vi "Image - Center and Zoom.vi"(8 "Error In":errorcluster, 10 "Image Data":T2, 11 "Pict Refnum":refnum<vi>) -> (0 "Error Out":errorcluster, 2 "Rect Out":T1, 3 "new picture":picture)   [LabVIEW 2020]
uses:
  <vilib>/picture/picture.llb/imagedata.ctl
  <vilib>/Utility/miscctls.llb/LVPointTypeDef.ctl
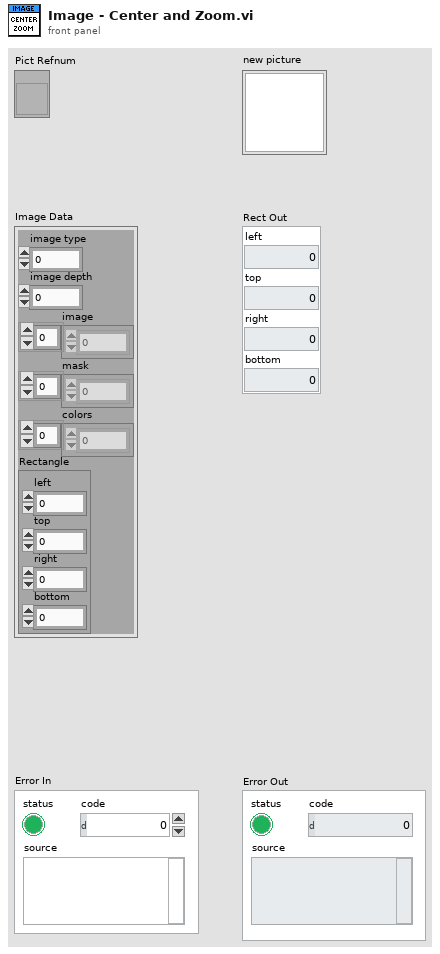
[diagram p1: front panel]
types:
  T1 = cluster{"left":i16, "top":i16, "right":i16, "bottom":i16}
  T2 = typedef "imagedata.ctl" = cluster{"image type":i32, "image depth":i32, "image":u8[], "mask":u8[], "colors":u32[], "Rectangle":cluster{"left":i16, "top":i16, "right":i16, "bottom":i16}}
  T3 = typedef "LVPointTypeDef.ctl" = cluster{"Horizontal":i16, "Vertical":i16}
  T4 = typedef "LVBoundsTypeDef.ctl" = cluster{"Width":u32, "Height":u32}
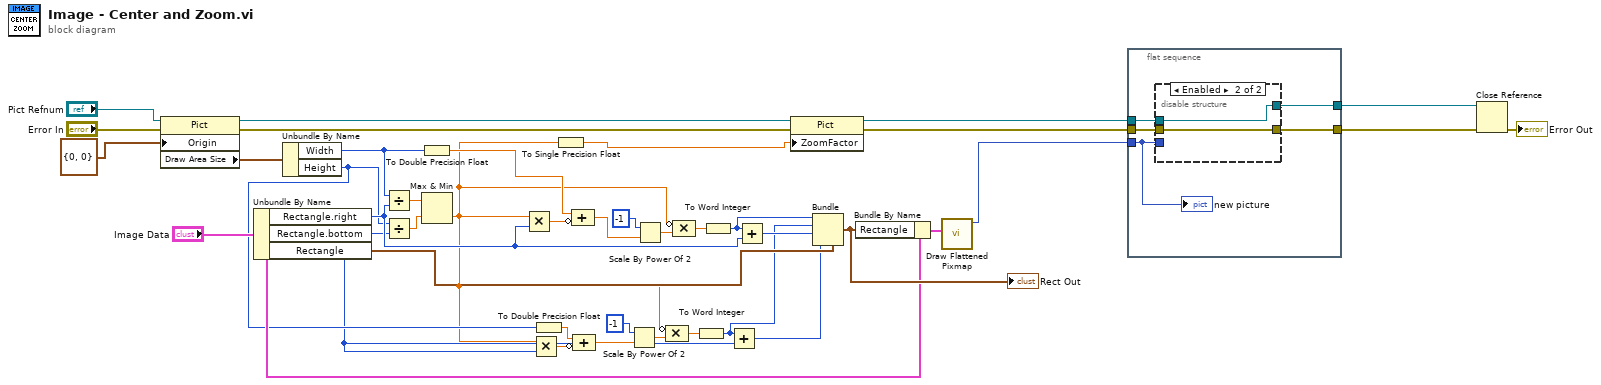
[diagram p0: block diagram]
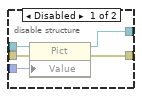
[diagram p2: hidden frame]
diagram:
  n1 = property class="Pict"(reference="Pict Refnum", error in="Error In", "Origin"=T3 {"Horizontal"=0, "Vertical"=0}) -> (reference out=w16:refnum<vi>, error out=w39:errorcluster, "Draw Area Size"=w17:T4)
  n2 = Unbundle By Name("Image Data") -> ("Rectangle.right"=w27:i16, "Rectangle.bottom"=w6:i16, "Rectangle"=w31:T1)
  n3 = Unbundle By Name(w17) -> ("Width"=w21:u32, "Height"=w7:u32)
  n4 = Divide(x=w21, y=w27) -> (x/y=w34:dbl)
  n5 = Divide(x=w7, y=w6) -> (x/y=w35:dbl)
  n6 = To Double Precision Float(number=w21) -> (double precision float=w32:dbl)
  n7 = Max & Min(x=w34, y=w35) -> (min(x,y)=w2:dbl)  [unwired: 1 out]
  n8 = Multiply(x=w2, y=w27) -> (x*y=w26:dbl)
  n9 = Multiply(x=w2, y=w6) -> (x*y=w13:dbl)
  n10 = To Double Precision Float(number=w7) -> (double precision float=w12:dbl)
  n11 = To Single Precision Float(number=w2) -> (single precision float=w1:sgl)
  n12 = Compound Arithmetic op=ADD(w32, invert w26) -> (w25:dbl)
  n13 = Compound Arithmetic op=ADD(w12, invert w13) -> (w8:dbl)
  n14 = Scale By Power Of 2(n=i16 -1, x=w8) -> (x*2^n=w10:dbl)
  n15 = Scale By Power Of 2(n=i16 -1, x=w25) -> (x*2^n=w24:dbl)
  n16 = Compound Arithmetic op=MULTIPLY(invert w2, w10) -> (w11:dbl)
  n17 = Compound Arithmetic op=MULTIPLY(invert w2, w24) -> (w23:dbl)
  n18 = To Word Integer(number=w11) -> (16bit integer=w5:i16)
  n19 = To Word Integer(number=w23) -> (16bit integer=w22:i16)
  n20 = Add(x=w5, y=w6) -> (x+y=w4:i16)
  n21 = Add(x=w22, y=w27) -> (x+y=w30:i16)
  n22 = property class="Pict"(reference=w16, error in=w39, "ZoomFactor"=w1) -> (reference out=w14:refnum<vi>, error out=w38:errorcluster)
  n23 = Bundle(cluster=w31, "left"=w22, "top"=w5, "right"=w30, "bottom"=w4) -> (w29:T1)
  "Rect Out" <- w29
  n24 = Bundle By Name(cluster="Image Data", "Rectangle"=w29) -> (w28:T2)
  n25 = call <vilib>:"Draw Flattened Pixmap.vi"("image data"=w28) -> ("new picture"=w15:picture)  [unwired: 8 in]
  n26 = flat-sequence {
    tunnel: w38 -> [w45]
    tunnel: [w44] -> w36
    tunnel: w15 -> [w41]
    tunnel: w14 -> [w43]
    tunnel: [w42] -> w3
    frame #0 {
      n27 = disable-structure shown="Enabled" {
        disable-tunnel: w45 -> [w50 w52]
        disable-tunnel: [w49 w52] -> w44
        disable-tunnel: w43 -> [w48 w51]
        disable-tunnel: [w47 w51] -> w42
        disable-tunnel: w41 -> [w46 _]
        frame Disabled {
          n28 = property class="Pict"(reference=w48, error in=w50, "Value"=w46) -> (reference out=w47:refnum<vi>, error out=w49:errorcluster)
        }
        frame Enabled {
        }
      }
      "new picture" <- w41
    }
  }
  n29 = Close Reference(reference=w3, error in (no error)=w36) -> (error out=→"Error Out":errorcluster)
